vi "Variant to Type Info.vi"(6 "Py-Object Type Signature":T3, 8 "error in (no error)":errorcluster, 11 "Type":variant) -> (0 "error out":errorcluster, 3 "Type Info":T1)   [LabVIEW 2020, in "G-Embedded-Python-Interpreter-Toolkit.lvlib"]
uses:
  G-Embedded-Python-Interpreter-Toolkit.lvlib
  <vilib>/Utility/Data Type/Type Definitions/Type Definition Info.ctl
  Type Information.ctl
  <vilib>/Utility/Data Type/Type Definitions/Data Type.ctl
  8cdebbe9-3e59-4fbe-97b0-695fa0ebc24d.vi
  <vilib>/Utility/error.llb/Error Cluster From Error Code.vi
  <vilib>/Comparison/Equal/Equal Functor/Equal Functor.lvclass
  <vilib>/Utility/Data Type/NI_Data Type.lvlib
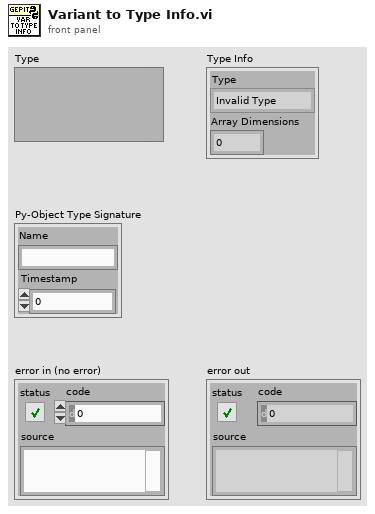
[diagram p1: front panel]
types:
  T1 = typedef "G-Embedded-Python-Interpreter-Toolkit.lvlib/Type Information.ctl" = cluster{"Type":T2, "Array Dimensions":u8}
  T2 = typedef "NI_Data Type.lvlib/Data Type.ctl" = enum8{"Invalid Type", "Void", "I8", "I16", "I32", "I64", "U8", "U16", "U32", "U64", "Single Float", "Double Float", "Extended Float", "Single Complex", "Double Complex", "Extended Complex", "Enum U8", "Enum U16", "Enum U32", "Enum U64", "Single Float With Unit", "Double Float With Unit", "Extended Float With Unit", "Single Complex with Unit", "Double Complex with Unit", "Extended Complex with Unit", "Boolean", "String", "Path", "Picture", "Tag", "Array", "Cluster", "Variant", "LV Variant", "Waveform", "Timestamp", "Digital Waveform", "Digital Data", "ExpressData", "Refnum", "External Data", "VI", "Poly VI", "LabVIEW Class Instance", "Fixed Point", "Set Collection", "Map Collection"}
  T3 = typedef "NI_Data Type.lvlib/Type Definition Info.ctl" = cluster{"Name":string, "Timestamp":u32}
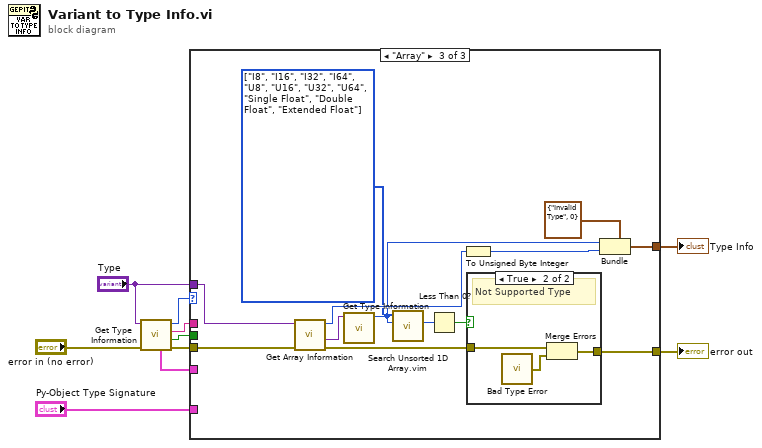
[diagram p0: block diagram]
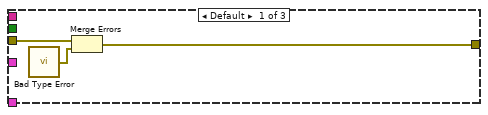
[diagram p2: hidden frame]
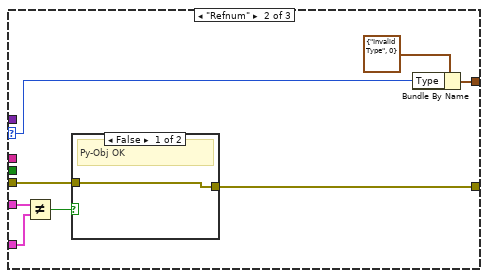
[diagram p3: hidden frame]
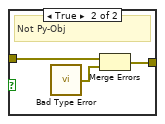
[diagram p4: hidden frame]
diagram:
  n1 = call <vilib>:"Get Type Information.vi"("error in (no error)"="error in (no error)", "variant"="Type") -> ("error out"=w4:errorcluster, "type definition"=w6:bool, "name"=w5:string, "type"=w1:T2, "type definition info"=w7:T3)  [unwired: 5 in]
  n2 = case shown="\"Array\"" w1 {
    selector: w1 -> [_ w17 _]
    tunnel: "Type" -> [_ _ w38]
    tunnel: [_ w18 w35] -> w2
    tunnel: w4 -> [w11 w15 w34]
    tunnel: [w13 w14 w28] -> w9
    tunnel: w5 -> [_ _ _]
    tunnel: w6 -> [_ _ _]
    tunnel: w7 -> [_ w21 _]
    tunnel: "Py-Object Type Signature" -> [_ w20 _]
    frame Default {
      n3 = call "Bad Type Error.vi"() -> ("Unsupported Type Error"=w12:errorcluster)
      n4 = Merge Errors(w11, w12) -> (w13:errorcluster)
    }
    frame "Refnum" {
      n5 = Not Equal?(x=w21, y=w20) -> (x != y?=w16:bool)
      n6 = case shown="False" w16 {
        tunnel: w15 -> [w22 w24]
        tunnel: [w22 w23] -> w14
        frame False {
          # "Py-Obj OK"
        }
        frame True {
          # "Not Py-Obj"
          n7 = call "Bad Type Error.vi"() -> ("Unsupported Type Error"=w25:errorcluster)
          n8 = Merge Errors(w24, w25) -> (w23:errorcluster)
        }
      }
      n9 = Bundle By Name(cluster=T1 {"Type"=enum."Invalid Type", "Array Dimensions"=0} ("Type Info"), "Type"=w17) -> (w18:T1)
    }
    frame "Array" {
      w26 = T2[] [enum."I8", enum."I16", enum."I32", enum."I64", enum."U8", enum."U16", enum."U32", enum."U64", enum."Single Float", enum."Double Float", enum."Extended Float"] items=["Invalid Type", "Void", "I8", "I16", "I32", "I64", "U8", "U16", "U32", "U64", "Single Float", "Double Float", "Extended Float", "Single Complex", "Double Complex", "Extended Complex", "Enum U8", "Enum U16", "Enum U32", "Enum U64", "Single Float With Unit", "Double Float With Unit", "Extended Float With Unit", "Single Complex with Unit", "Double Complex with Unit", "Extended Complex with Unit", "Boolean", "String", "Path", "Picture", "Tag", "Array", "Cluster", "Variant", "LV Variant", "Waveform", "Timestamp", "Digital Waveform", "Digital Data", "ExpressData", "Refnum", "External Data", "VI", "Poly VI", "LabVIEW Class Instance", "Fixed Point", "Set Collection", "Map Collection"] ("type")
      n10 = call <vilib>:"Get Array Information.vi"("error in (no error)"=w34, "variant"=w38) -> ("error out"=w27:errorcluster, "array element data type"=w33:variant, "number of dimensions"=w37:i32)  [unwired: 6 in, 1 out]
      n11 = call <vilib>:"Get Type Information.vi"("variant"=w33) -> ("type"=w31:T2)  [unwired: 6 in, 4 out]
      n12 = call "Search Unsorted 1D Array.vim"("element"=w31, "unsorted 1D array"=w26) -> ("index of element"=w30:i32)  [unwired: 9 in]
      n13 = Less Than 0?(x=w30) -> (x < 0?=w29:bool)
      n14 = To Unsigned Byte Integer(number=w37) -> (unsigned 8bit integer=w36:u8)
      n15 = case shown="True" w29 {
        tunnel: [w39 w40] -> w28
        tunnel: w27 -> [w39 w42]
        frame False {
          # "Type OK"
        }
        frame True {
          # "Not Supported Type"
          n16 = call "Bad Type Error.vi"() -> ("Unsupported Type Error"=w41:errorcluster)
          n17 = Merge Errors(w42, w41) -> (w40:errorcluster)
        }
      }
      n18 = Bundle(cluster=T1 {"Type"=enum."Invalid Type", "Array Dimensions"=0} ("Type Info"), "Type"=w31, "Array Dimensions"=w36) -> (w35:T1)
    }
  }
  "error out" <- w9
  "Type Info" <- w2
